vi "Saturate.vi"(9 "Max":sgl, 10 "Min":sgl, 11 "X in":dbl) -> (3 "X out":dbl)   [LabVIEW 2014]
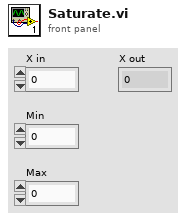
[diagram p1: front panel]
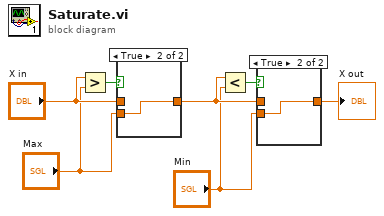
[diagram p0: block diagram]
diagram:
  n1 = Greater?(x="X in", y="Max") -> (0:w1:bool)
  n2 = case shown="True" w1 {
    tunnel: "Max" -> [_ w9]
    tunnel: [w8 w9] -> w6
    tunnel: "X in" -> [w8 _]
    frame False {
    }
    frame True {
    }
  }
  n3 = Less?(x=w6, y="Min") -> (x < y?=w4:bool)
  n4 = case shown="True" w4 {
    tunnel: "Min" -> [_ w11]
    tunnel: w6 -> [w10 _]
    tunnel: [w10 w11] -> w7
    frame False {
    }
    frame True {
    }
  }
  "X out" <- w7
